vi "_PC_NS_Wfm_Set_WaveformData.vi"(5 "wfm stop bool":refnum<k21>, 8 "error In":errorcluster, 9 "WfmData_U64 in":u64[](array[numeric]), 11 "writer name In":refnum<k21>) -> (0 "error Out":errorcluster, 3 "writer name Out":refnum<k21>)   [LabVIEW 2018]
uses:
  <vilib>/Platform/TimedLoop/XDataNode/timing_clust.ctl
  <vilib>/Platform/TimedLoop/XDataNode/nitl_modes.ctl
  <vilib>/Platform/TimedLoop/XDataNode/wakeup.ctl
  <vilib>/Platform/TimedLoop/XDataNode/XDataNode.xnode
  <vilib>/Platform/TimedLoop/XDataNode/XDNodeRunTimeDep.lvlib
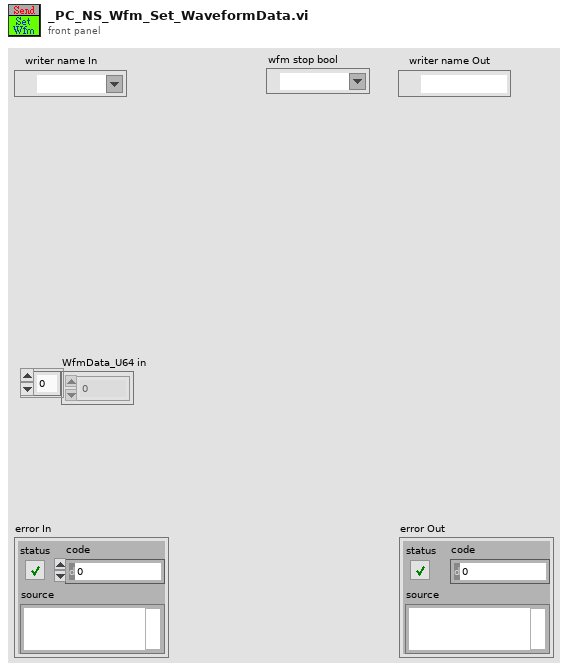
[diagram p1: front panel]
types:
  T1 = typedef "XDNodeRunTimeDep.lvlib/timing_clust.ctl" = cluster{"Expected End [f-1]":u64, "Actual End [f-1]":u64, "Finished Late? [f-1]":bool, "Expected End [i-1]":u64, "Actual End [i-1]":u64, "Finished Late? [i-1]":bool, "Expected Start [i]":u64, "Actual Start [i]":u64, "Expected Start [f]":u64, "Actual Start [f]":u64, "Source Name":string, "Structure Name":string, "Period":i64, "Deadline":i64, "Offset":i64, "Start":i64, "Priority":i32, "Timeout":i32, "Mode":T2, "Wakeup Reason":T3, "Error":errorcluster, "Source Type":string, "Secondary Source Type":string, "Global End Time":u64, "Global Start Time":u64, "Frame Duration":u64, "Iteration Duration":u64, "Assigned CPU":i32, "I/O Scan Engine Mode":u32}
  T2 = typedef "XDNodeRunTimeDep.lvlib/nitl_modes.ctl" = enum32{"No Change", "Process missed periods, maintain original phase", "Discard missed periods, maintain original phase", "Process missed periods, ignore original phase", "Discard missed periods, ignore original phase"}
  T3 = typedef "XDNodeRunTimeDep.lvlib/wakeup.ctl" = enum32{"Normal", "Aborted", "Asynchronous wakeup", "Timing source error", "Timed loop error", "Timeout"}
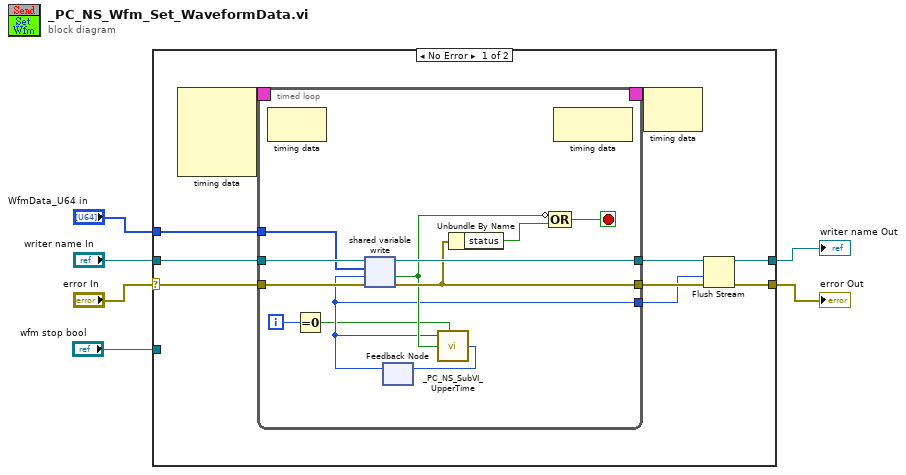
[diagram p0: block diagram]
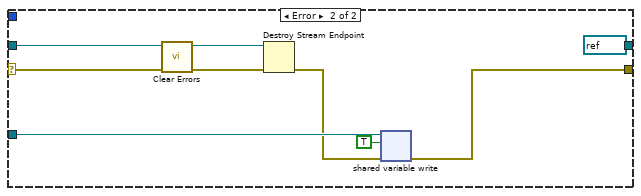
[diagram p2: hidden frame]
diagram:
  n1 = case shown="No Error" "error In" {
    selector: "error In" -> [w7 w40]
    tunnel: "writer name In" -> [w16 w39]
    tunnel: [w9 w33] -> w3
    tunnel: "WfmData_U64 in" -> [w15 _]
    tunnel: [w10 refnum<k21> refnum ("writer name")] -> w2
    tunnel: "wfm stop bool" -> [_ w36]
    frame No Error {
      n2 = node-c288() -> (w12:T1)  [unwired: 4 in]
      n3 = timed-loop {
        tunnel: w16 -> [w28]
        tunnel: w7 -> [w27]
        tunnel: [w26] -> w14
        tunnel: [w24] -> w13
        tunnel: w15 -> [w21]
        timing: w12 -> [_]
        timing-out: [_] -> w11
        tunnel: [w19] -> w8
        i -> [w18]
        stop <- w22 stop-if-true
        n4 = node-c288() -> ()  [unwired: 1 in, 1 out]
        n5 = Equal To 0?(x=w18) -> (x = 0?=w17:bool)
        n6 = feedback #1() -> (w19:i32)  [unwired: 1 in]
        n7 = shared-variable-write(w28, w27, w21, w19) -> (w26:refnum<k21>, w24:errorcluster, w23:bool)
        n8 = call "_PC_NS_SubVI_UpperTime.vi"("Init Time"=w19, "Init? (F)"=w17, "Update (T)"=w23) -> ("UpdateTime"=w20:i32)  [unwired: 2 in]
        n9 = feedback-in #1(w20) -> ()
        n10 = Unbundle By Name(w24) -> ("status"=w25:bool)
        n11 = Compound Arithmetic op=OR(invert w23, w25) -> (w22:bool)
        n12 = node-c288() -> ()  [unwired: 1 in, 1 out]
      }
      n13 = node-c288(w11) -> ()  [unwired: 1 out]
      n14 = Flush Stream(8:w13, 9:w8, 11:w14) -> (0:w9:errorcluster, 3:w10:refnum<k21>)  [unwired: 1 in, 1 out]
    }
    frame Error {
      n15 = call <vilib>:"Clear Errors.vi"("error in (no error)"=w40) -> ("error out"=w38:errorcluster)  [unwired: 5 in, 1 out]
      n16 = Destroy Stream Endpoint(8:w38, 11:w39) -> (0:w35:errorcluster)
      n17 = shared-variable-write(w36, w35, TRUE ("data in")) -> (w33:errorcluster)  [unwired: 1 out]
    }
  }
  "error Out" <- w3
  "writer name Out" <- w2
